vi "Re-Center Motor.vi"(9 "Desired offset from switch":dbl=-500.0 format="%.2f") -> (2 "Must move":dbl, 3 "Current Position":dbl format="%.2f")   [LabVIEW 2010]
panel:
  out "String":string
  out "sine offset size":string
  out "concatenated string":string
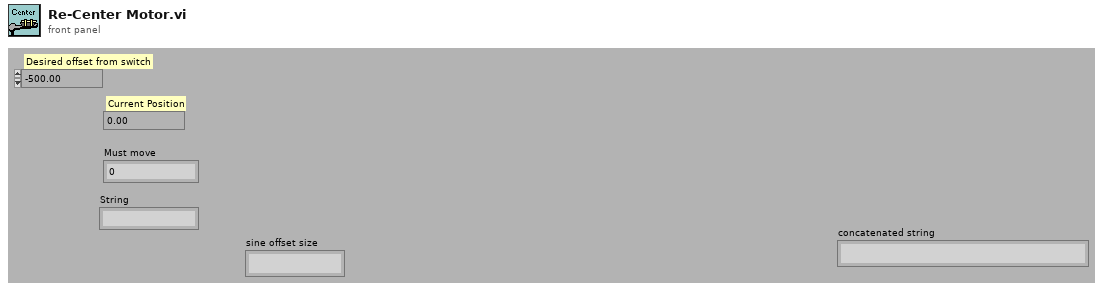
[diagram p1: front panel]
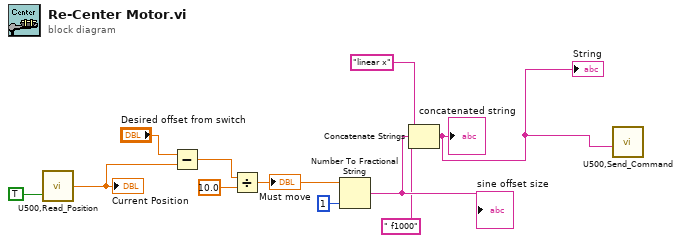
[diagram p0: block diagram]
diagram:
  n1 = call "U500,Read_Position.vi"("Auto Update"=TRUE) -> ("Position"=w9:dbl)  [unwired: 1 in]
  "Current Position" <- w9
  n2 = Subtract(x="Desired offset from switch", y=w9) -> (x-y=w8:dbl)
  n3 = Divide(x=w8, y=10.0) -> (x/y=w2:dbl)
  "Must move" <- w2
  n4 = Number To Fractional String(number=w2, precision (6)=i16 1) -> (F-format string=w4:string)  [unwired: 2 in]
  "sine offset size" <- w4
  n5 = Concatenate Strings("linear x" ("Command String"), w4, " f1000" ("string")) -> (w1:string)
  "concatenated string" <- w1
  "String" <- w1
  n6 = call "U500,Send_Command.vi"("Command String"=w1) -> ()  [unwired: 9 in, 2 out]
